vi "Perform Action.vi"(8 "error in":errorcluster, 10 "Input":variant, 11 "Virt Instrument Base in":refnum<class "Virt DAQmx DC Generator.lvclass">) -> (0 "error out":errorcluster, 2 "Output":variant, 3 "Virt Instrument Base out":refnum<class "Virt DAQmx DC Generator.lvclass">)   [LabVIEW 2023, in "Virt Instrs AO.lvlib" / "Virt DAQmx DC Generator.lvclass"]
uses:
  Virt DAQmx DC Generator.lvclass
  Virt Instr Host/Virt Instr Local.lvclass/Virt Instr Local.ctl
  Virt Instr Base/Virt Instr Base.lvclass/Virt Instr Base.ctl
  Virt DAQmx DC Generator.lvclass/Virt DAQmx DC Generator.ctl
  Virt Instr Host/Virt Instr Local.lvclass
  Instrument/Instrument.lvclass
  Virt Instr Base/Virt Instr Base.lvclass
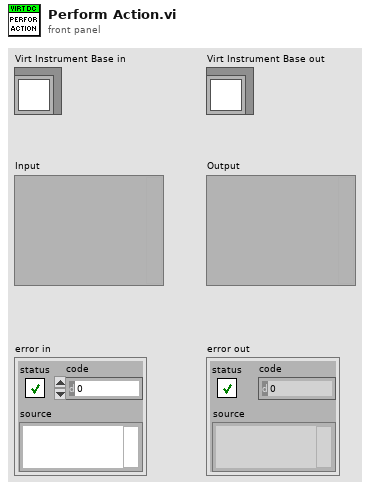
[diagram p1: front panel]
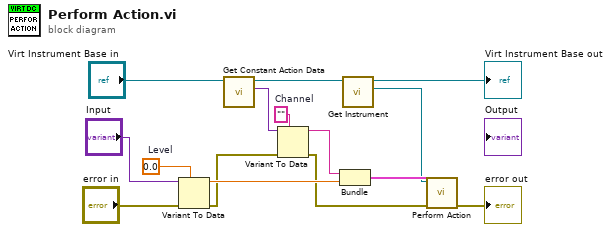
[diagram p0: block diagram]
diagram:
  w8 = 0.0  # Level
  w14 = ""  # Channel
  n1 = Variant To Data(error in="error in", type=w8, Variant="Input") -> (data=w15:dbl, error out=w6:errorcluster)
  n2 = call "Get Constant Action Data.vi"("Virt Instr Base in"="Virt Instrument Base in") -> ("Constant Action Data"=w11:variant, "Virt Instr Base out"=w12:refnum<class "Virt DAQmx DC Generator.lvclass">)  [unwired: 9 in]
  n3 = Variant To Data(error in=w6, type=w14, Variant=w11) -> (data=w13:string, error out=w7:errorcluster)
  n4 = Bundle("Channel"=w13, "Level"=w15) -> (w10:cluster{"Channel":string, "Level":dbl})  [unwired: 1 in]
  n5 = call "Get Instrument.vi"("Virt Instr Base in"=w12) -> ("HAL GOOP4.lvlib:Instrument"=w9:refnum<class "Instrument.lvclass">, "Virt Instr Base out"=→"Virt Instrument Base out":refnum<class "Virt DAQmx DC Generator.lvclass">)  [unwired: 9 in]
  n6 = call "Perform Action.vi"("Error In"=w7, "Input"=w10, "reference in"=w9) -> ("Error Out"=→"error out":errorcluster)  [unwired: 6 in, 2 out]
